vi "Apply.vi"(8 "error in":errorcluster, 11 "AO DAQmx DC Simulated CFG in":refnum<class "AO DAQmx DC CFG Simulated.lvclass">) -> (0 "error out":errorcluster, 3 "AO DAQmx DC Simulated CFG out":refnum<class "AO DAQmx DC CFG Simulated.lvclass">)   [LabVIEW 2024, in "DAQmx Simulated CFGs.lvlib" / "AO DAQmx DC CFG Simulated.lvclass"]
uses:
  AO DAQmx DC CFG Simulated.lvclass
  Configurations/CFG Base/CFG Base.lvclass/CFG Base.ctl
  AO DAQmx DC CFG/AO DAQmx DC CFG.lvclass
  Configurations/CFG Base/CFG Base.lvclass
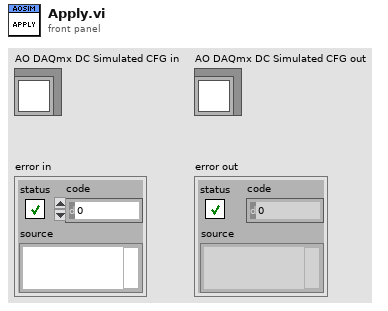
[diagram p1: front panel]
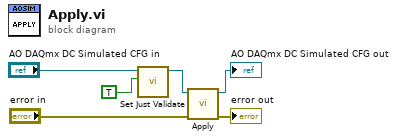
[diagram p0: block diagram]
diagram:
  n1 = call "Set Just Validate.vi"("Just Validate"=TRUE, "CFG Base in"="AO DAQmx DC Simulated CFG in") -> ("CFG Base out"=w2:refnum<class "AO DAQmx DC CFG Simulated.lvclass">)  [unwired: 9 in]
  n2 = call-parent "Apply.vi"("error in"="error in", "AO DAQmx DC CFG in"=w2) -> ("error out"=→"error out":errorcluster, "AO DAQmx DC CFG out"=→"AO DAQmx DC Simulated CFG out":refnum<class "AO DAQmx DC CFG Simulated.lvclass">)  [unwired: 8 in]
